vi "Voltage - Continuous HW Timed Output.vi"() -> ()   [LabVIEW 2014]
doc: "This example demonstrates how to continuously re-generate analog output data from a buffer in your computer's memory.\n\nRefer to your device documentation for pinouts and hardware capabilities."
uses:
  <vilib>/Utility/error.llb/DialogType.ctl
  <vilib>/DAQmx/create/channels.llb/DAQmx Create Channel (AO-Voltage-Basic).vi
  <vilib>/DAQmx/configure/timing.llb/DAQmx Timing (Sample Clock).vi
  <vilib>/DAQmx/write.llb/DAQmx Write (Analog 1D Wfm NChan NSamp).vi
  <resource>/objmgr/daqmx.rc
  <vilib>/measure/NI_MABase.lvlib
panel:
  in  "Output Array":T1(array[cluster])=[{"Waveform Type"=0, "Amplitude"=1.0, "Frequency"=10.0}] {"Frequency" format="%0.2p"; "Amplitude" format="%0.2p"; "Waveform Type" items=["Sine Wave", "Triangle Wave", "Square Wave", "Sawtooth Wave"]}
  in  "Number of Samples":i32=1000
  in  "Stop":bool
  out "Waveform Graph":waveform(dbl)[](graph)=[{"t0"=timestamp(0 s since 1904-01-01), "dt"=0.001, "Y"=[]}]
  in  "Sample Rate":dbl=1000.0
  in  "Sample Clock Source":tag="OnboardClock"
  in  "Max Voltage":dbl=5.0
  in  "Min Voltage":dbl=-5.0
  in  "Physical Channel(s)":tag="Dev1/ao0"
  out "Actual Sample Rate":dbl=1000.0 format="%0.2f"
  # "Channel Settings"
  # "Output"
  # "Timing and Buffer Settings"
  # "Waveform Settings"
  # "The number of elements in the waveform array must equal the number of channels in the task."
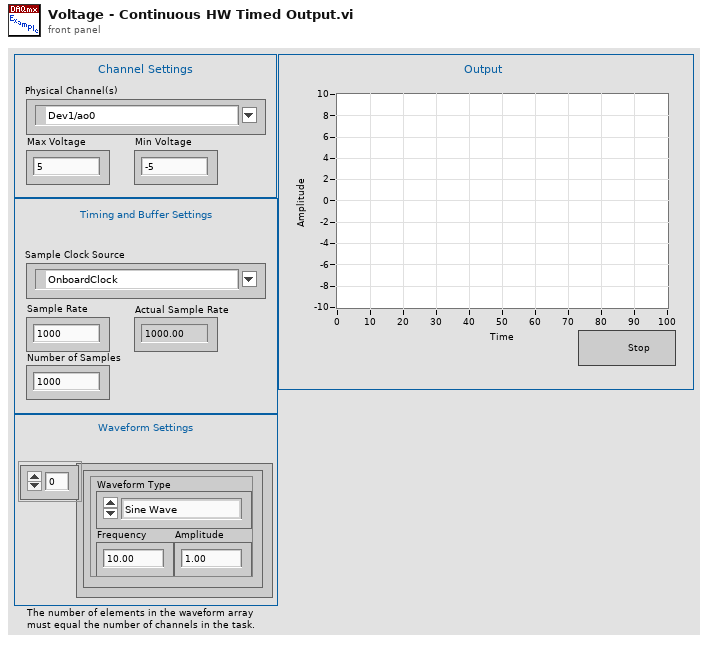
[diagram p1: front panel]
types:
  T1 = cluster{"Waveform Type":u16, "Amplitude":dbl, "Frequency":dbl}[]
  T2 = typedef "DialogType.ctl" = u16
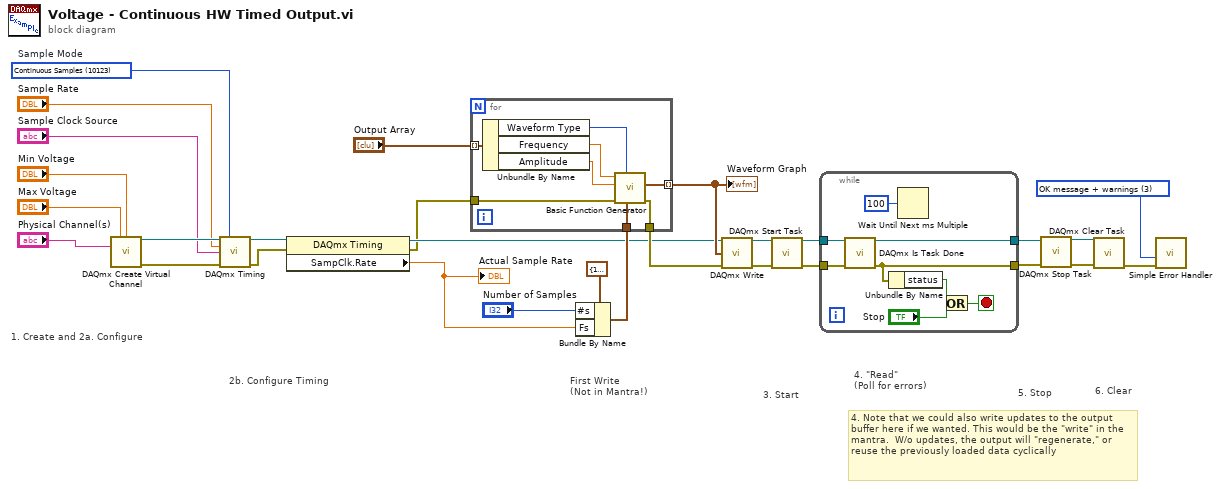
[diagram p0: block diagram]
diagram:
  w5 = T2 3 items=["no dialog", "OK message", "continue or stop message", "OK message + warnings", "continue/stop + warnings"] ("type of dialog (OK msg:1)")
  w27 = 10123 items=["Finite Samples"=10178, "Continuous Samples"=10123, "Hardware Timed Single Point"=12522]  # Sample Mode
  # "6. Clear"
  # "5. Stop"
  # "4. Note that we could also write updates to the output buffer here if we wanted. This would be the \"write\" in the mantra.  W/o updates, the output will \"regenerate,\" or reuse the previously loaded data cyclically"
  # "4. \"Read\"\n(Poll for errors)"
  # "3. Start"
  # "First Write\n(Not in Mantra!)"
  # "2b. Configure Timing"
  # "1. Create and 2a. Configure"
  n1 = call-poly <vilib>:"DAQmx Create Virtual Channel.vi"("maximum value"="Max Voltage", "minimum value"="Min Voltage", "physical channels"="Physical Channel(s)") -> ("task out"=w25:refnum<k21>, "error out"=w26:errorcluster)  [unwired: 11 in]
  n2 = call-poly <vilib>:"DAQmx Timing.vi"("task/channels in"=w25, "sample mode"=w27, "rate"="Sample Rate", "source"="Sample Clock Source", "error in"=w26) -> ("task out"=w29:refnum<k21>, "error out"=w28:errorcluster)  [unwired: 9 in]
  n3 = property class="DAQmx Timing"(reference=w29, error in=w28) -> (reference out=w4:refnum<k21>, error out=w3:errorcluster, "SampClk.Rate"=w16:dbl)
  "Actual Sample Rate" <- w16
  n4 = Bundle By Name(cluster=cluster{"Fs":dbl, "#s":dbl} {"Fs"=1000.0, "#s"=1000.0} ("sampling info"), "#s"="Number of Samples", "Fs"=w16) -> (w15:cluster{"Fs":dbl, "#s":dbl})
  n5 = for {
    tunnel: w3 -> [w37]
    tunnel: w15 -> [w36]
    tunnel: [w35] -> w12
    tunnel: "Output Array" -> [w34] mode=indexing
    tunnel: [w30] -> w10 mode=indexing
    n6 = Unbundle By Name(w34) -> ("Waveform Type"=w33:u16, "Frequency"=w32:dbl, "Amplitude"=w31:dbl)
    n7 = call <vilib>:"Basic Function Generator.vi"("sampling info"=w36, "signal type"=w33, "error in (no error)"=w37, "amplitude"=w31, "frequency"=w32) -> ("error out"=w35:errorcluster, "signal out"=w30:waveform(dbl))  [unwired: 4 in, 1 out]
  }
  "Waveform Graph" <- w10
  n8 = call-poly <vilib>:"DAQmx Write.vi"("task/channels in"=w4, "data"=w10, "error in"=w12) -> ("task out"=w14:refnum<k21>, "error out"=w13:errorcluster)  [unwired: 10 in, 1 out]
  n9 = call <vilib>:"DAQmx Start Task.vi"("task/channels in"=w14, "error in"=w13) -> ("task out"=w24:refnum<k21>, "error out"=w23:errorcluster)  [unwired: 12 in]
  n10 = while {
    tunnel: w24 -> [w45]
    tunnel: w23 -> [w44]
    tunnel: [w41] -> w6
    tunnel: [w42] -> w7
    stop <- w43 stop-if-true
    n11 = call <vilib>:"DAQmx Is Task Done.vi"("task/channels in"=w45, "error in"=w44) -> ("task out"=w42:refnum<k21>, "error out"=w41:errorcluster)  [unwired: 11 in, 1 out]
    n12 = Unbundle By Name(w41) -> ("status"=w40:bool)
    n13 = Wait Until Next ms Multiple(millisecond multiple=u32 100) -> ()  [unwired: 1 out]
    n14 = Or(x=w40, y="Stop") -> (x .or. y?=w43:bool)
  }
  n15 = call <vilib>:"DAQmx Stop Task.vi"("task/channels in"=w7, "error in"=w6) -> ("task out"=w9:refnum<k21>, "error out"=w8:errorcluster)  [unwired: 12 in]
  n16 = call <vilib>:"DAQmx Clear Task.vi"("task in"=w9, "error in"=w8) -> ("error out"=w22:errorcluster)  [unwired: 13 in]
  n17 = call <vilib>:"Simple Error Handler.vi"("type of dialog (OK msg:1)"=w5, "error in (no error)"=w22) -> ()  [unwired: 3 in, 5 out]
